vi "Get-mapping-offset.vi"(8 "error in":errorcluster, 11 "Data ref. in":refnum<data-value>) -> (0 "error IO":errorcluster, 2 "Start offset":dbl caption="Start offset [s]", 3 "Data ref.":refnum<data-value>)   [LabVIEW 2013, in "CameraVision.lvlib" / "CV-Main.lvclass"]
uses:
  CV-Main.lvclass
  CV-Main.lvclass/CV-Main.ctl
  Mapping/CV-Mapping.lvclass/CV-Mapping.ctl
  Read Mapping params.vi
  Mapping/Read Start off-set.vi
  Mapping/CV-Mapping.lvclass
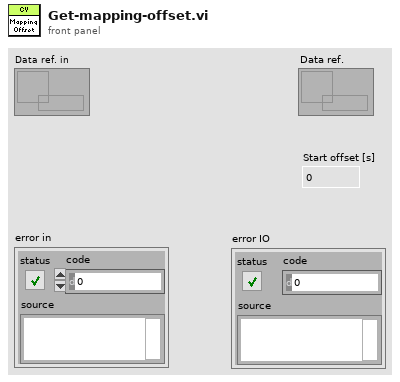
[diagram p1: front panel]
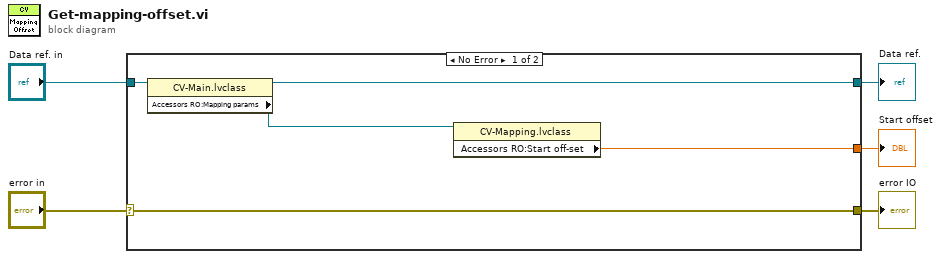
[diagram p0: block diagram]
diagram:
  n1 = case shown="No Error" "error in" {
    selector: "error in" -> [w8 w12]
    tunnel: "Data ref. in" -> [w10 w11]
    tunnel: [w8 w12] -> w3
    tunnel: [w9 w11] -> w2
    tunnel: [w7 _] -> w1
    frame No Error {
      n2 = property class="CV-Main.lvclass"(reference=w10) -> (reference out=w9:refnum<data-value>, "Accessors RO:Mapping params"=w6:refnum<data-value>)  [unwired: 1 in, 1 out]
      n3 = property class="CV-Mapping.lvclass"(reference=w6) -> ("Accessors RO:Start off-set"=w7:dbl)  [unwired: 1 in, 2 out]
    }
    frame Error {
    }
  }
  "error IO" <- w3
  "Data ref." <- w2
  "Start offset" <- w1
